vi "server stats buffer.vi"(4 "Server Stats in":T1={"scan rate"=10.0, "# connections"=0, "channel settings"=[]} {"channel settings"."lower input limits" format="%.4f"; "channel settings"."upper input limits" format="%.4f"; "scan rate" format="%.2f"}, 6 "# connections":i32, 7 "state":enum16{"write", "read", "change connections"}(ring)) -> (0 "Server Stats out":T1={"scan rate"=10.0, "# connections"=0, "channel settings"=[]} {"channel settings"."lower input limits" format="%.4f"; "channel settings"."upper input limits" format="%.4f"; "scan rate" format="%.2f"})   [LabVIEW 2019]
uses:
  Server stats.ctl
panel:
  # "Hz"
  # "Hz"
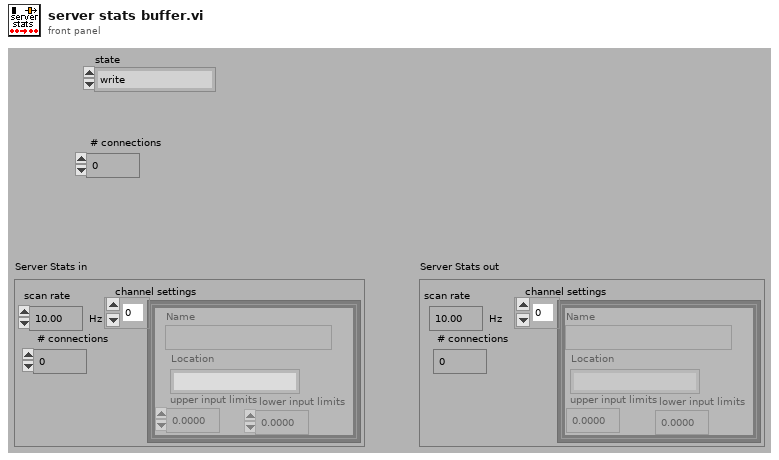
[diagram p1: front panel]
types:
  T1 = typedef "Server stats.ctl" = cluster{"scan rate":dbl, "# connections":i32, "channel settings":cluster{"Name":string, "upper input limits":sgl, "lower input limits":sgl, "Location":string}[]}
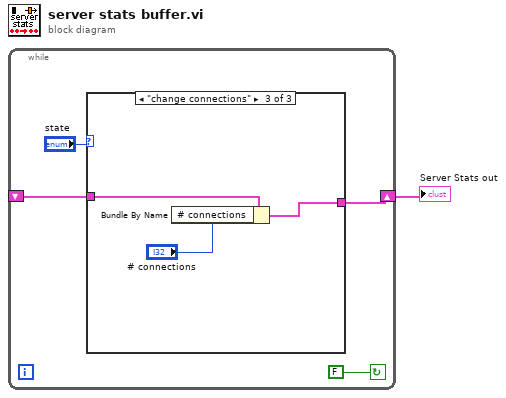
[diagram p0: block diagram]
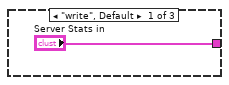
[diagram p2: hidden frame]
diagram:
  n1 = while {
    shift-right: [w4] -> w1
    shift-left: _ -> [w3]
    stop <- FALSE continue-if-true
    n2 = case shown="\"change connections\"" "state" {
      tunnel: ["Server Stats in" w7 w9] -> w4
      tunnel: w3 -> [_ w7 w10]
      frame "write", Default {
      }
      frame "read" {
      }
      frame "change connections" {
        n3 = Bundle By Name(cluster=w10, "# connections"="# connections") -> (w9:T1)
      }
    }
  }
  "Server Stats out" <- w1
